vi "variable1.vi"() -> ()   [LabVIEW 2025]
panel:
  in  "affiche":bool
  out "Slide 2":dbl(slide) scale=0.0..10.0
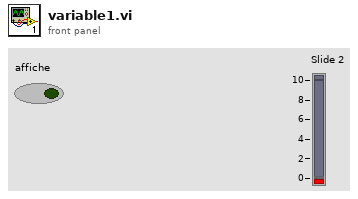
[diagram p1: front panel]
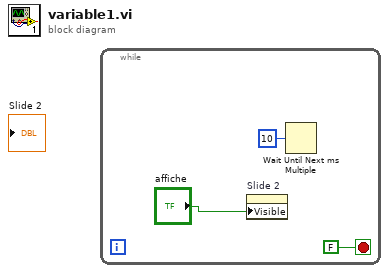
[diagram p0: block diagram]
diagram:
  n1 = while {
    stop <- FALSE stop-if-true
    n2 = property on="Slide 2" class="Slide (strict)"("Visible"="affiche") -> ()  [unwired: 2 in, 2 out]
    n3 = Wait Until Next ms Multiple(millisecond multiple=u32 10) -> ()  [unwired: 1 out]
  }
